vi "get_algs.vi"(8 "error in":errorcluster) -> (0 "error out":errorcluster, 3 "Available Algorithms":T1[](array[typedef]))   [LabVIEW 2013]
uses:
  TD Algorithm Information.ctl
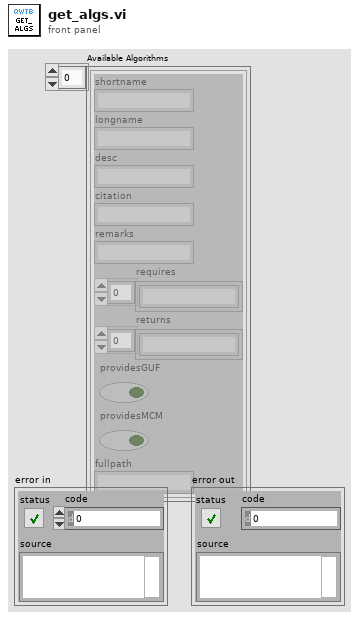
[diagram p1: front panel]
types:
  T1 = typedef "TD Algorithm Information.ctl" = cluster{"shortname":string, "longname":string, "desc":string, "citation":string, "remarks":string, "requires":string[], "returns":string[], "providesGUF":bool, "providesMCM":bool, "fullpath":string}
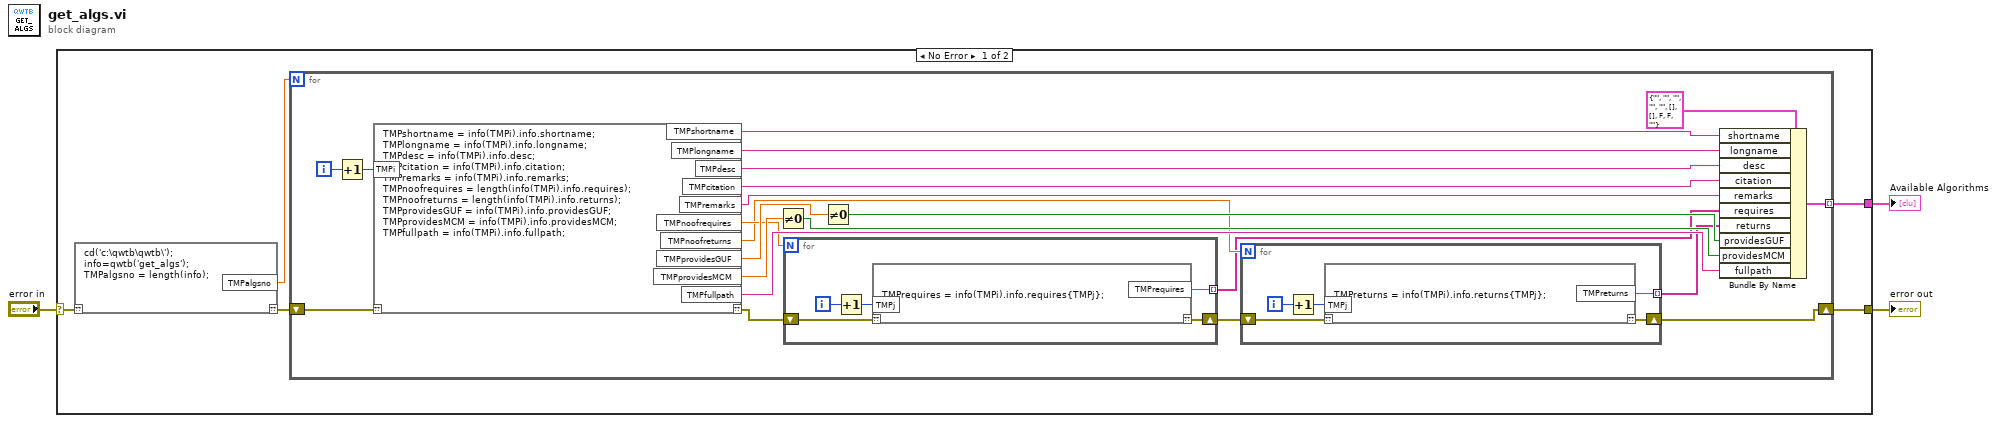
[diagram p0: block diagram]
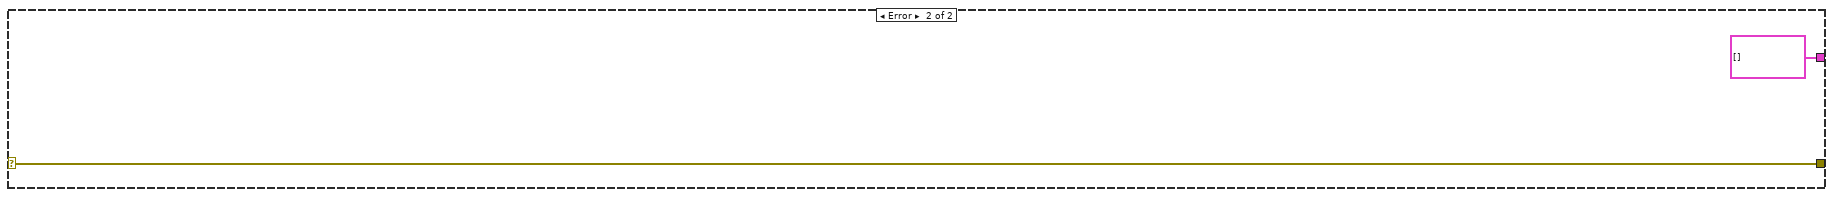
[diagram p2: hidden frame]
diagram:
  n1 = case shown="No Error" "error in" {
    selector: "error in" -> [w5 w42]
    tunnel: [w6 T1[] []] -> w3
    tunnel: [w4 w42] -> w1
    frame No Error {
      n2 = script code="cd('c:\\qwtb\\qwtb\\');\ninfo=qwtb('get_algs');\nTMPalgsno = length(info);"("??"=w5) -> ("??"=w7:errorcluster, "TMPalgsno"=w8:dbl)
      n3 = for {
        N: w8 -> [_]
        tunnel: [w24] -> w6 mode=indexing
        shift-right: [w12] -> w4
        shift-left: w7 -> [w30]
        i -> [w16]
        n4 = Increment(x=w16) -> (x+1=w17:i32)
        n5 = script code="TMPshortname = info(TMPi).info.shortname;\nTMPlongname = info(TMPi).info.longname;\nTMPdesc = info(TMPi).info.desc;\nTMPcitation = info(TMPi).info.citation;\nTMPremarks = info(TMPi).info.remarks;\nTMPnoofrequires = length(info(TMPi).info.requires);\nTMPnoofreturns = length(info(TMPi).info.returns);\nTMPprovidesGUF = info(TMPi).info.providesGUF;\nTMPprovidesMCM = info(TMPi).info.providesMCM;\nTMPfullpath = info(TMPi).info.fullpath;"("??"=w30, "TMPi"=w17) -> ("??"=w15:errorcluster, "TMPshortname"=w28:string, "TMPlongname"=w27:string, "TMPdesc"=w26:string, "TMPfullpath"=w25:string, "TMPnoofrequires"=w14:dbl, "TMPnoofreturns"=w11:dbl, "TMPcitation"=w18:string, "TMPremarks"=w19:string, "TMPprovidesGUF"=w21:dbl, "TMPprovidesMCM"=w23:dbl)
        n6 = Not Equal To 0?(x=w23) -> (x != 0?=w22:bool)
        n7 = for {
          N: w14 -> [_]
          shift-right: [w37] -> w13
          shift-left: w15 -> [w40]
          tunnel: [w36] -> w10 mode=indexing
          i -> [w38]
          n8 = Increment(x=w38) -> (x+1=w39:i32)
          n9 = script code="TMPrequires = info(TMPi).info.requires{TMPj};"("??"=w40, "TMPj"=w39) -> ("??"=w37:errorcluster, "TMPrequires"=w36:string)
        }
        n10 = Not Equal To 0?(x=w21) -> (x != 0?=w20:bool)
        n11 = for {
          N: w11 -> [_]
          shift-right: [w32] -> w12
          shift-left: w13 -> [w35]
          tunnel: [w31] -> w9 mode=indexing
          i -> [w33]
          n12 = Increment(x=w33) -> (x+1=w34:i32)
          n13 = script code="TMPreturns = info(TMPi).info.returns{TMPj};"("??"=w35, "TMPj"=w34) -> ("??"=w32:errorcluster, "TMPreturns"=w31:string)
        }
        n14 = Bundle By Name(cluster=T1 {"shortname"="", "longname"="", "desc"="", "citation"="", "remarks"="", "requires"=[], "returns"=[], "providesGUF"=FALSE, "providesMCM"=FALSE, "fullpath"=""} ("Algorithm Information"), "shortname"=w28, "longname"=w27, "desc"=w26, "citation"=w18, "remarks"=w19, "requires"=w10, "returns"=w9, "providesGUF"=w20, "providesMCM"=w22, "fullpath"=w25) -> (w24:T1)
      }
    }
    frame Error {
    }
  }
  "Available Algorithms" <- w3
  "error out" <- w1
